vi "Oriantation Finish.vi"   [LabVIEW 2013]
types:
  T1 = typedef "WPI_AnalogChannelDevRef.ctl" = cluster{"DevStatus":errorcluster, "Analog Module":T2, "Analog Channel":T3}
  T2 = typedef "FPGA_TypedefAnalogModule.ctl" = enum16{"Analog Module 1", "Analog Module 2"}
  T3 = typedef "FPGA_AIChannel.ctl" = enum8{"AI 1", "AI 2", "AI 3", "AI 4", "AI 5", "AI 6", "AI 7", "AI 8", "Invalid"}
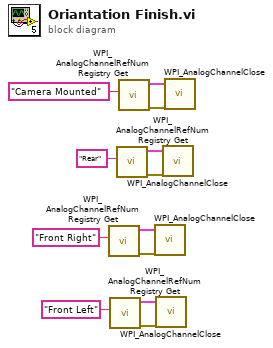
[diagram p0: block diagram]
diagram:
  n1 = call <vilib>:"WPI_AnalogChannelRefNum Registry Get.vi"("refnum name"="Front Right") -> ("error out"=w6:errorcluster, "AIDeviceRef"=w5:T1)  [unwired: 9 in]
  n2 = call <vilib>:"WPI_AnalogChannelRefNum Registry Get.vi"("refnum name"="Front Left") -> ("error out"=w1:errorcluster, "AIDeviceRef"=w2:T1)  [unwired: 9 in]
  n3 = call <vilib>:"WPI_AnalogChannelRefNum Registry Get.vi"("refnum name"="Rear") -> ("error out"=w7:errorcluster, "AIDeviceRef"=w8:T1)  [unwired: 9 in]
  n4 = call <vilib>:"WPI_AnalogChannelRefNum Registry Get.vi"("refnum name"="Camera Mounted") -> ("error out"=w12:errorcluster, "AIDeviceRef"=w11:T1)  [unwired: 9 in]
  n5 = call <vilib>:"WPI_AnalogChannelClose.vi"("error in (no error)"=w6, "AIDeviceRef"=w5) -> ()  [unwired: 9 in, 1 out]
  n6 = call <vilib>:"WPI_AnalogChannelClose.vi"("error in (no error)"=w1, "AIDeviceRef"=w2) -> ()  [unwired: 9 in, 1 out]
  n7 = call <vilib>:"WPI_AnalogChannelClose.vi"("error in (no error)"=w7, "AIDeviceRef"=w8) -> ()  [unwired: 9 in, 1 out]
  n8 = call <vilib>:"WPI_AnalogChannelClose.vi"("error in (no error)"=w12, "AIDeviceRef"=w11) -> ()  [unwired: 9 in, 1 out]
